vi "Validate Incoming Packet.vi"(8 "error in (no error)":errorcluster, 10 "ControlPacket":refnum<class "ControlPacket.lvclass">, 11 "Session.Client in":refnum<class "Session.Client.lvclass">) -> (0 "error out":errorcluster, 2 "ControlPacket out":refnum<class "ControlPacket.lvclass">, 3 "Session.Client out":refnum<class "Session.Client.lvclass">)   [LabVIEW 2013, in "MQTT Client.lvlib" / "Session.Client.lvclass"]
uses:
  Session.Client.lvclass
  <vilib>/LabVIEW Open Source Project/MQTT Control Packets/Control Packets/ControlPacket/ControlPacket.lvclass
  <vilib>/LabVIEW Open Source Project/MQTT Connection/MQTT_Base/Session/Session.lvclass
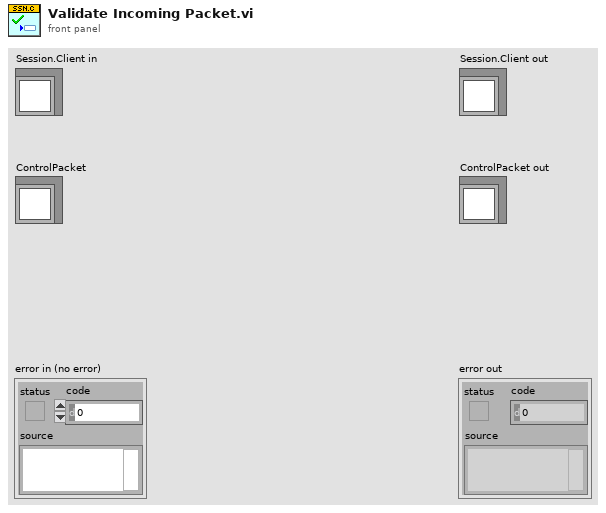
[diagram p1: front panel]
types:
  T1 = typedef "MQTT_Control_Packets.lvlib/ControlPacket.lvclass/Control Packet Type -- enum.ctl" = enum16{"Reserved", "CONNECT", "CONNACK", "PUBLISH", "PUBACK", "PUBREC", "PUBREL", "PUBCOMP", "SUBSCRIBE", "SUBACK", "UNSUBSCRIBE", "UNSUBACK", "PINGREQ", "PINGRESP", "DISCONNECT", "AUTH"}
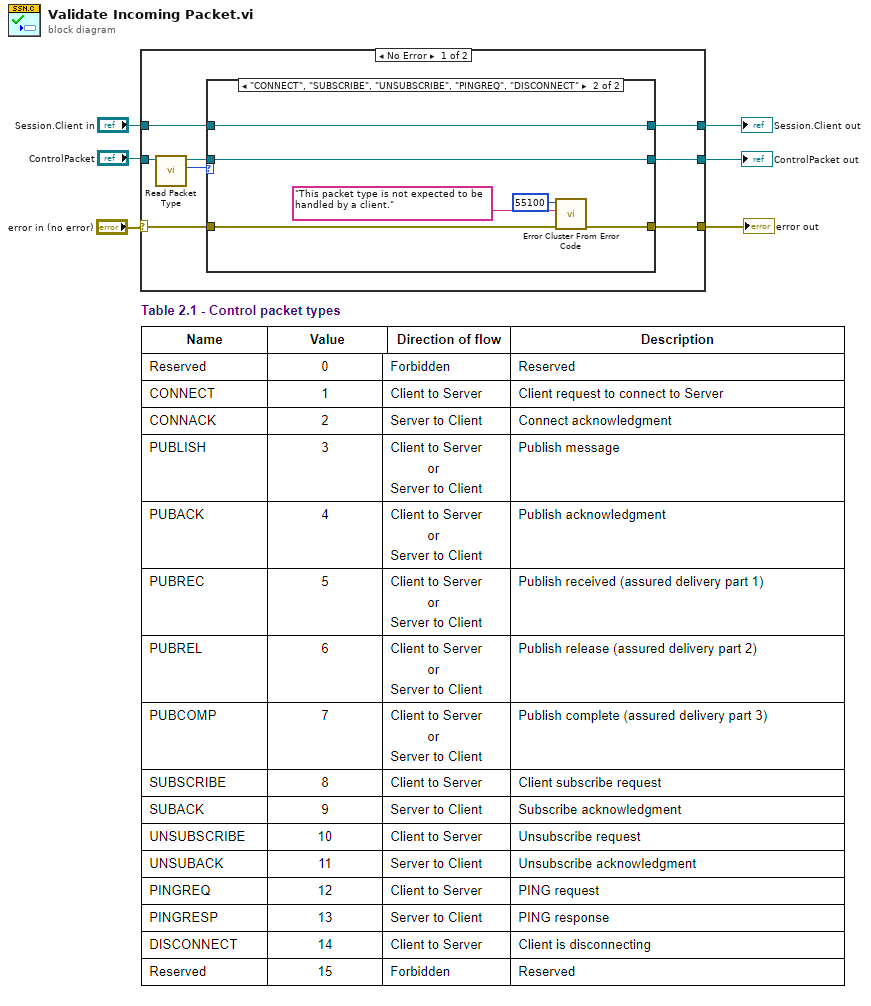
[diagram p0: block diagram]
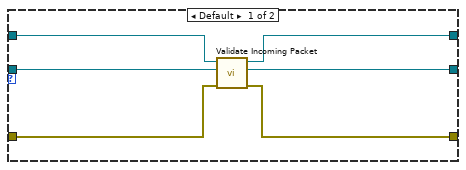
[diagram p2: hidden frame]
diagram:
  n1 = case shown="No Error" "error in (no error)" {
    selector: "error in (no error)" -> [w12 w29]
    tunnel: [w11 w29] -> w1
    tunnel: [w8 w28] -> w3
    tunnel: "Session.Client in" -> [w7 w28]
    tunnel: "ControlPacket" -> [w13 w27]
    tunnel: [w14 w27] -> w2
    frame No Error {
      n2 = call <vilib>:"Read Packet Type.vi"("ControlPacket in"=w13) -> ("Control Packet Type"=w9:T1, "ControlPacket out"=w10:refnum<class "ControlPacket.lvclass">)  [unwired: 9 in]
      n3 = case shown="\"CONNECT\", \"SUBSCRIBE\", \"UNSUBSCRIBE\", \"PINGREQ\", \"DISCONNECT\"" w9 {
        tunnel: w10 -> [w18 w21]
        tunnel: [w17 w21] -> w14
        tunnel: w12 -> [w16 w24]
        tunnel: [w15 w22] -> w11
        tunnel: [w19 w23] -> w8
        tunnel: w7 -> [w20 w23]
        frame Default {
          n4 = call-parent "Validate Incoming Packet.vi"("error in (no error)"=w16, "ControlPacket"=w18, "Session in"=w20) -> ("error out"=w15:errorcluster, "ControlPacket out"=w17:refnum<class "ControlPacket.lvclass">, "Session out"=w19:refnum<class "Session.Client.lvclass">)  [unwired: 6 in]
        }
        frame "CONNECT", "SUBSCRIBE", "UNSUBSCRIBE", "PINGREQ", "DISCONNECT" {
          n5 = call <vilib>:"Error Cluster From Error Code.vi"("error in (no error)"=w24, "error message (\"\")"="This packet type is not expected to be handled by a client.", "error code (0)"=55100) -> ("error out"=w22:errorcluster)  [unwired: 6 in]
        }
      }
    }
    frame Error {
    }
  }
  "error out" <- w1
  "Session.Client out" <- w3
  "ControlPacket out" <- w2
